vi "Get Page Configuration.vi"(10 "Page Number":i32, 11 "Page Configurations":T2(array[cluster])) -> (3 "Plot Channel Configurations":T1[](array[typedef]))   [LabVIEW 2017, in "DTacq Plot Display Library.lvlib"]
uses:
  DTacq Plot Display Library.lvlib
  Typedefs/Plot Channel Configruation--Cluster.ctl
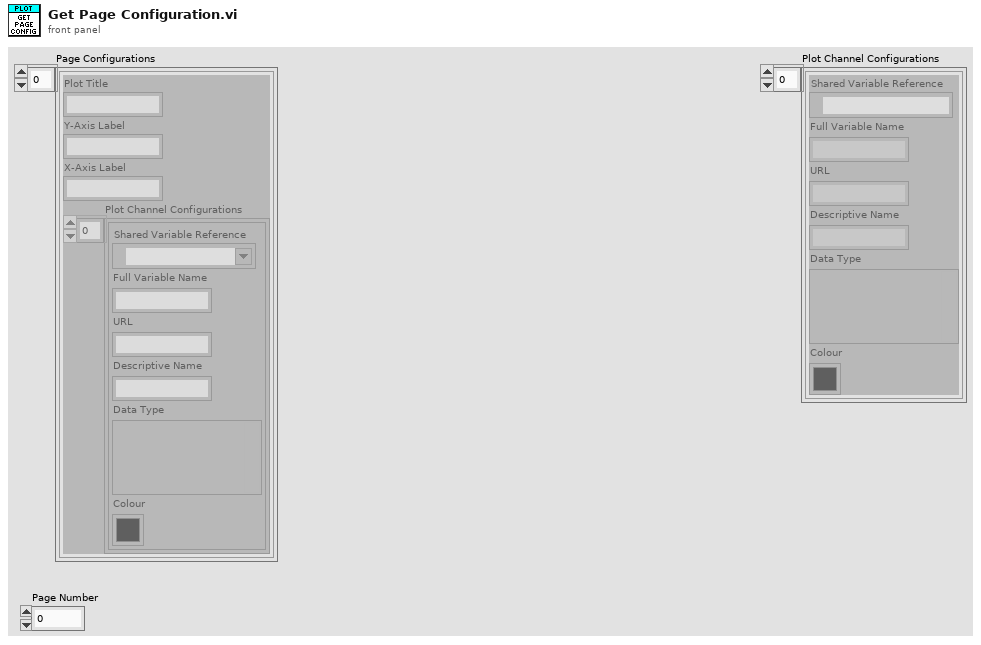
[diagram p1: front panel]
types:
  T1 = typedef "DTacq Plot Display Library.lvlib/Plot Channel Configruation--Cluster.ctl" = cluster{"Shared Variable Reference":refnum<k21>, "Full Variable Name":string, "URL":string, "Descriptive Name":string, "Data Type":variant, "Colour":u32}
  T2 = cluster{"Plot Title":string, "Y-Axis Label":string, "X-Axis Label":string, "Plot Channel Configurations":T1[]}[]
  T3 = cluster{"Plot Title":string, "Y-Axis Label":string, "X-Axis Label":string, "Plot Channel Configurations":T1[]}
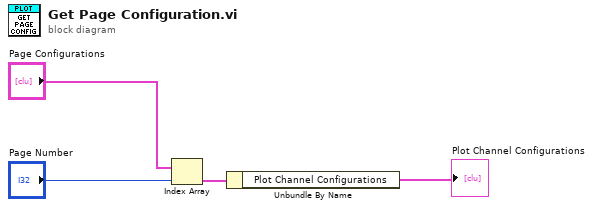
[diagram p0: block diagram]
diagram:
  n1 = Index Array(array="Page Configurations", index="Page Number") -> (element=w3:T3)
  n2 = Unbundle By Name(w3) -> ("Plot Channel Configurations"=→"Plot Channel Configurations":T1[])
